vi "GEA2 HEWH ERDs.vi"(7 "Enable Diagnostic Data":T1, 8 "Error In":errorcluster, 9 "Disable ERD (Main)":bool, 10 "LV Program":T2, 11 "Disable Electronic Mixing Valve (EMV) List":bool) -> (0 "Error Out":errorcluster, 1 "Read ERD List":T4[](array[typedef]) {"ERD Number" format="%.0x"}, 2 "GEA Inputs":T3 {"Destination" format="%.0x"; "Source" format="%.0x"}, 3 "ERD Headers":string[](array[string]))   [LabVIEW 2016]
uses:
  type defs/ERD Read Data In.ctl
  type defs/Data Type.ctl
  type defs/Source_Destination.ctl
  Save File/File Setup (Public)/Type Definition/Save File DOE LabView Program.ctl
  Washer HCC/Washer HCC NEWFI/Type Definitions/HCC Washer Types.ctl
  <vilib>/Utility/error.llb/whitespace.ctl
  library/GEA2_Toolkit.lvlib
  Save File/File Setup.lvlib
panel:
  in  "Tab Control":enum32{"HEWH", "Washer"}(tab)
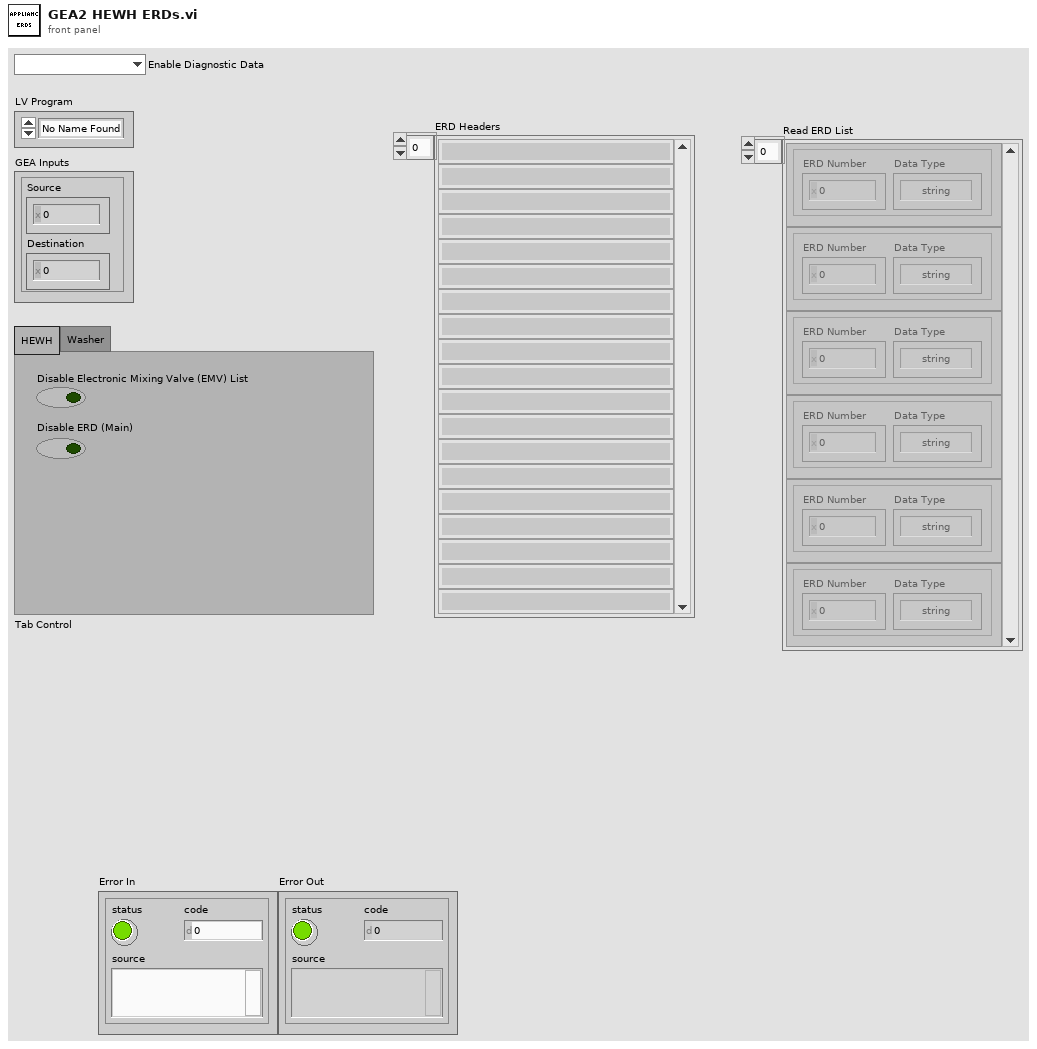
[diagram p1: front panel]
types:
  T1 = typedef "HCC Washer Types.ctl" = enum16{"", "Viper Washer", "Hawk Washer", "2015 Washer", "2017 Washer"}
  T2 = typedef "File Setup.lvlib/Save File DOE LabView Program.ctl" = enum16{"No Name Found", "DOE Stand", "Dishwasher Kitchen", "Portable Stand", "HEWH", "Dryer", "Dryer WILT", "HCC", "PRAT", "HEWH RLT", "Refrigeration"}
  T3 = typedef "GEA2_Toolkit.lvlib/Source_Destination.ctl" = cluster{"Source":u8, "Destination":u8}
  T4 = typedef "GEA2_Toolkit.lvlib/ERD Read Data In.ctl" = cluster{"ERD Number":u16, "Data Type":T5}
  T5 = typedef "GEA2_Toolkit.lvlib/Data Type.ctl" = enum16{"string", "boolean", "uint8_t", "uint16_t", "uint32_t", "uint64_t"}
  T6 = typedef "whitespace.ctl" = u16
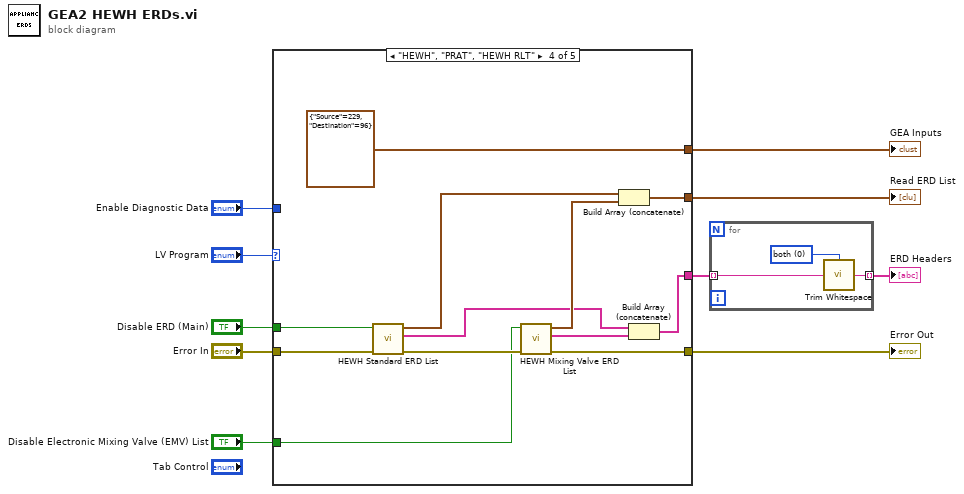
[diagram p0: block diagram]
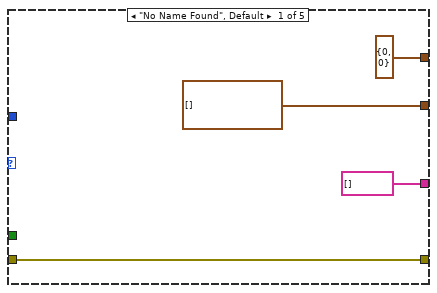
[diagram p2: hidden frame]
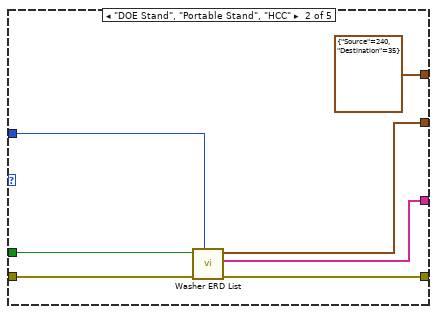
[diagram p3: hidden frame]
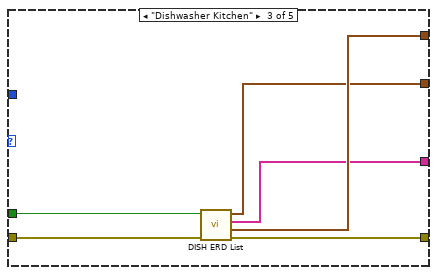
[diagram p4: hidden frame]
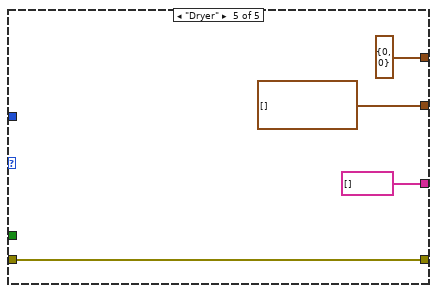
[diagram p5: hidden frame]
diagram:
  n1 = case shown="\"HEWH\", \"PRAT\", \"HEWH RLT\"" "LV Program" {
    tunnel: [string[] [] w21 w26 w37 string[] []] -> w5
    tunnel: [T4[] [] ("Read ERD List") w20 w25 w34 T4[] [] ("Read ERD List")] -> w6
    tunnel: [T3 {"Source"=0, "Destination"=0} ("GEA Inputs") T3 {"Source"=240, "Destination"=35} ("GEA Inputs") w27 T3 {"Source"=229, "Destination"=96} ("GEA Inputs") T3 {"Source"=0, "Destination"=0} ("GEA Inputs")] -> w10
    tunnel: [w14 w16 w22 w38 w42] -> w9
    tunnel: "Error In" -> [w14 w17 w23 w30 w42]
    tunnel: "Disable ERD (Main)" -> [_ w19 w24 w33 _]
    tunnel: "Enable Diagnostic Data" -> [_ w15 _ _ _]
    tunnel: "Disable Electronic Mixing Valve (EMV) List" -> [_ _ _ w28 _]
    frame "No Name Found", Default {
    }
    frame "DOE Stand", "Portable Stand", "HCC" {
      n2 = call "Washer ERD List.vi"("Enable Diagnostic Data"=w15, "Error In"=w17, "Disable ERD (Main)"=w19) -> ("Error Out"=w16:errorcluster, "Header Array"=w21:string[], "Read ERD List"=w20:T4[])  [unwired: 6 in]
    }
    frame "Dishwasher Kitchen" {
      n3 = call "DISH ERD List.vi"("Error In"=w23, "Disable ERD (Main)"=w24) -> ("Error Out"=w22:errorcluster, "GEA Inputs"=w27:T3, "Array"=w26:string[], "Read ERD List"=w25:T4[])  [unwired: 6 in]
    }
    frame "HEWH", "PRAT", "HEWH RLT" {
      n4 = call "HEWH Standard ERD List.vi"("Error In"=w30, "Disable ERD (Main)"=w33) -> ("Error Out"=w29:errorcluster, "Header"=w31:string[], "Read ERD List"=w32:T4[])  [unwired: 7 in]
      n5 = call "HEWH Mixing Valve ERD List.vi"("error in (no error)"=w29, "Disable Electronic Mixing Valve (EMV) List"=w28) -> ("error out"=w38:errorcluster, "Headers"=w36:string[], "Read ERD List"=w35:T4[])  [unwired: 7 in]
      n6 = Build Array (concatenate)(w32, w35) -> (w34:T4[])
      n7 = Build Array (concatenate)(w31, w36) -> (w37:string[])
    }
    frame "Dryer" {
    }
  }
  "Read ERD List" <- w6
  "GEA Inputs" <- w10
  "Error Out" <- w9
  n8 = for {
    tunnel: w5 -> [w45] mode=indexing
    tunnel: [w44] -> w4 mode=indexing
    w46 = T6 0 items=["both", "start of string", "end of string"] ("location (both)")
    n9 = call <vilib>:"Trim Whitespace.vi"("string"=w45, "location (both)"=w46) -> ("trimmed string"=w44:string)
  }
  "ERD Headers" <- w4
